vi "DrawFullBackground.vi"(8 "error in (no error)":errorcluster, 11 "Menu in":refnum<class "Menu.lvclass">) -> (0 "error out":errorcluster, 3 "Menu out":refnum<class "Menu.lvclass">)   [LabVIEW 2019, in "RT_Game.lvlib" / "Menu.lvclass"]
uses:
  Menu.lvclass
  C:/Users/FreshBob/Dropbox/VIs/myRIO_GameConsole/RT/RT_Game/Game/Game.lvclass
  Game/Game.lvclass
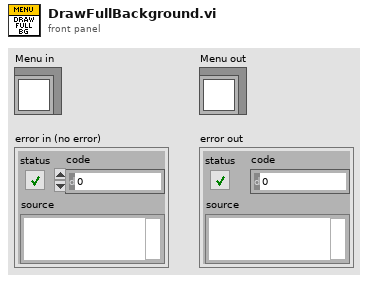
[diagram p1: front panel]
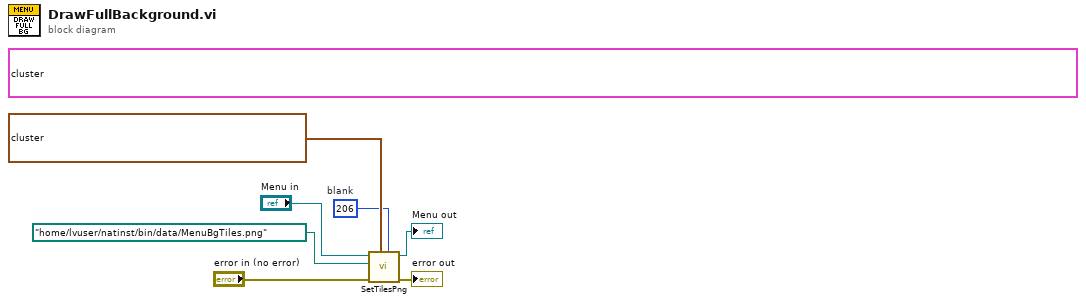
[diagram p0: block diagram]
diagram:
  w1 = u32 206  # blank
  (unwired) cluster{"Color":fxp<+,3,3>, "TileCode":string}[] [{"Color"=0.0, "TileCode"="line_leftup"}, {"Color"=1.0, "TileCode"="line_vert"}, {"Color"=2.0, "TileCode"="line_rightdown"}, {"Color"=3.0, "TileCode"="line_rightup"}, {"Color"=4.0, "TileCode"="##replace-5-2"}, {"Color"=5.0, "TileCode"="line_leftdown"}, {"Color"=6.0, "TileCode"="line_hor"}, {"Color"=7.0, "TileCode"="bg1#replace-5-2"}] ("Tiles")
  n1 = call "SetTilesPng.vi"("DefaultTileCode"=w1, "Tiles"=cluster{"Color":fxp<+,3,3>, "TileCode":u32}[] [{"Color"=0.0, "TileCode"=1073741905}, {"Color"=1.0, "TileCode"=1073741908}, {"Color"=2.0, "TileCode"=1073741840}, {"Color"=3.0, "TileCode"=1073741904}, {"Color"=4.0, "TileCode"=1543503897}, {"Color"=5.0, "TileCode"=1073741841}, {"Color"=6.0, "TileCode"=1073741909}, {"Color"=7.0, "TileCode"=1543503896}], "error in (no error)"="error in (no error)", "Path"=path "/home/lvuser/natinst/bin/data/MenuBgTiles.png", "Game in"="Menu in") -> ("error out"=→"error out":errorcluster, "Game out"=→"Menu out":refnum<class "Menu.lvclass">)  [unwired: 3 in, 2 out]
